vi "ControlRead.vi"(0 "Data input":T1, 1 "Selected Item":string[](array[string]), 5 "error in":errorcluster) -> (14 "Data output":T1, 19 "error out":errorcluster)   [LabVIEW 2017]
doc: "<B>This VI is used for getting the selelcted property type, value and index, and setting the control value.</B>"
uses:
  <vilib>/Utility/miscctls.llb/LVStringsAndValuesArrayTypeDef_U16.ctl
  API/Tree/SLSC Tree Control.lvlib
  <vilib>/JDP Science/JSONtext/JSONtext.lvlib
  cd6786a6-1ea5-437c-bd7d-10aa4f833b89.vi
  1b247805-81af-4051-83cb-4bfd180f6ea7.vi
  Ctrl/Property.ctl
  Ctrl/PhysicalChannel.ctl
  Ctrl/Bitfield.ctl
  Ctrl/Register.ctl
  Ctrl/ScaleType.ctl
  Ctrl/Scale.ctl
  Ctrl/EnumValue.ctl
  Ctrl/Enum.ctl
  Ctrl/Caps.ctl
  Ctrl/Data.ctl
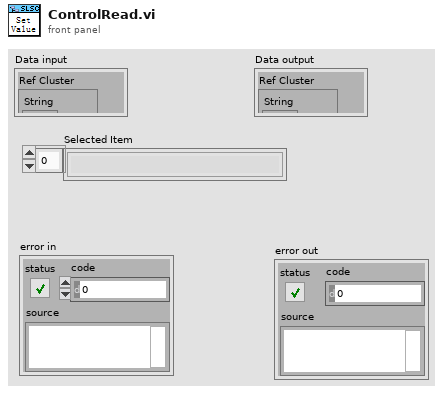
[diagram p1: front panel]
types:
  T1 = typedef "Data.ctl" = cluster{"Ref Cluster":cluster{"String":refnum<vi>, "U8":refnum<vi>, "I8":refnum<vi>, "U32":refnum<vi>, "I32":refnum<vi>, "U64":refnum<vi>, "I64":refnum<vi>, "Ring":refnum<vi>, "DBL":refnum<vi>, "Add":refnum<vi>, "Remove":refnum<vi>, "Property tree":refnum<vi>, "confirm":refnum<vi>}, "JSON Text":string, "Original JSON Text":string, "Caps":T2, "SLSC Output Tree":cluster{"Left Cell String":string, "Child Text":string[], "Child Tag":string, "Item Indent":i32, "Child Only?":bool, "Glyph Index":i32, "offline value":variant}[], "Ref Index and Control Type":cluster{"index":i32, "Datatype":string}, "Selected Type and name":cluster{"Selected Type":enum16{"Property", "Physical Channel", "Other"}, "Selected Property Name":string}, "Update whole Tree?":bool}
  T2 = typedef "Caps.ctl" = cluster{"properties":T3[], "physical channels":T4[], "registers":T5[], "scales":T7[], "enums":T9[], "productName":string}
  T3 = typedef "Property.ctl" = cluster{"name":string, "bitfield":string, "value":variant, "dataType":string, "min":variant, "max":variant, "scale":string, "access":string}
  T4 = typedef "PhysicalChannel.ctl" = cluster{"name":string, "properties":T3[]}
  T5 = typedef "Register.ctl" = cluster{"name":string, "address":i32, "size":i32, "bitfields":T6[], "initialValue":variant, "connectedProperties":string[]}
  T6 = typedef "Bitfield.ctl" = cluster{"name":string, "offset":i32, "size":i32, "signed":bool}
  T7 = typedef "Scale.ctl" = cluster{"name":string, "type":T8, "params":variant}
  T8 = typedef "ScaleType.ctl" = enum16{"NoScale", "Table", "Polynomial", "Linear"}
  T9 = typedef "Enum.ctl" = cluster{"name":string, "values":T10[]}
  T10 = typedef "EnumValue.ctl" = cluster{"name":string, "value":i32}
  T11 = enum16{"Show Selected Control", "All Visiable", "All Invisible"}
  T12 = cluster{"String":refnum<vi>, "U8":refnum<vi>, "I8":refnum<vi>, "U32":refnum<vi>, "I32":refnum<vi>, "U64":refnum<vi>, "I64":refnum<vi>, "Ring":refnum<vi>, "DBL":refnum<vi>, "Add":refnum<vi>, "Remove":refnum<vi>, "Property tree":refnum<vi>, "confirm":refnum<vi>}
  T13 = typedef "LVStringsAndValuesArrayTypeDef_U16.ctl" = cluster{"String":string, "Value":u16}[]
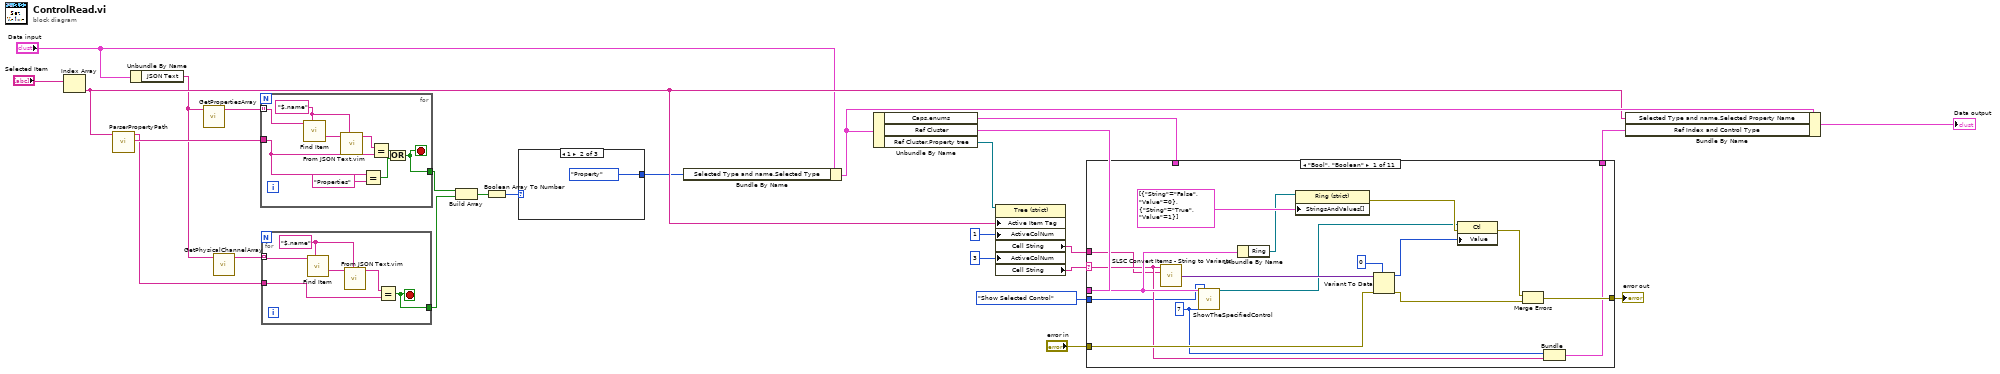
[diagram p0: block diagram]
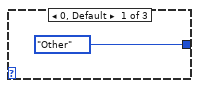
[diagram p2: hidden frame]
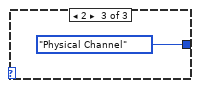
[diagram p3: hidden frame]
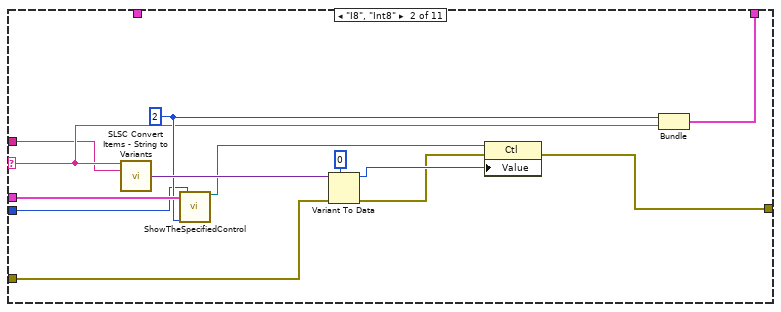
[diagram p4: hidden frame]
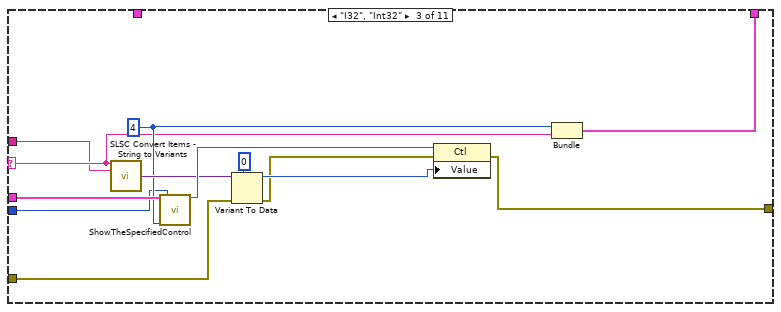
[diagram p5: hidden frame]
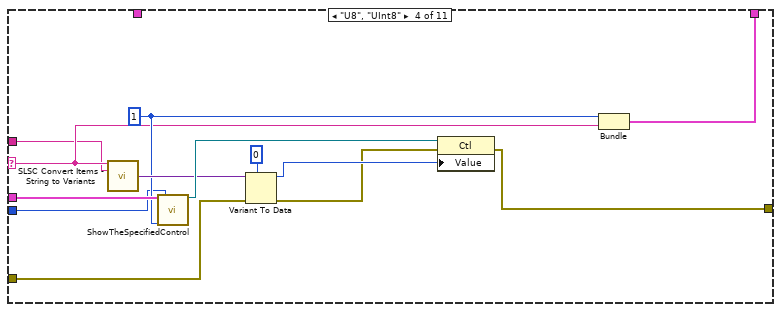
[diagram p6: hidden frame]
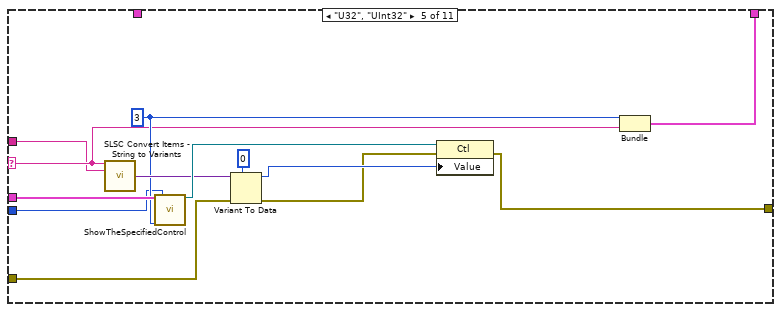
[diagram p7: hidden frame]
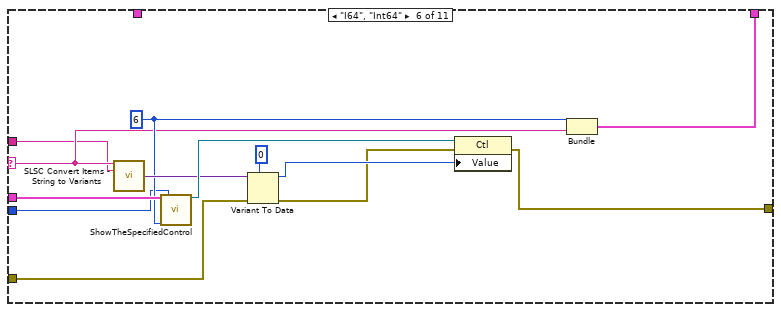
[diagram p8: hidden frame]
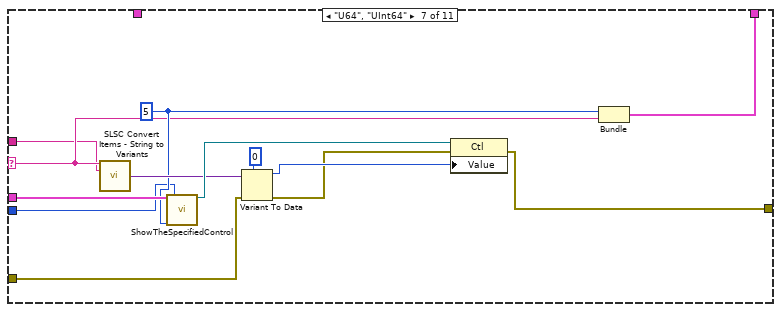
[diagram p9: hidden frame]
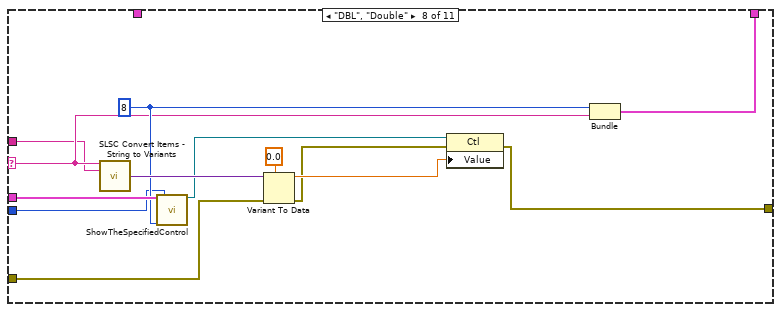
[diagram p10: hidden frame]
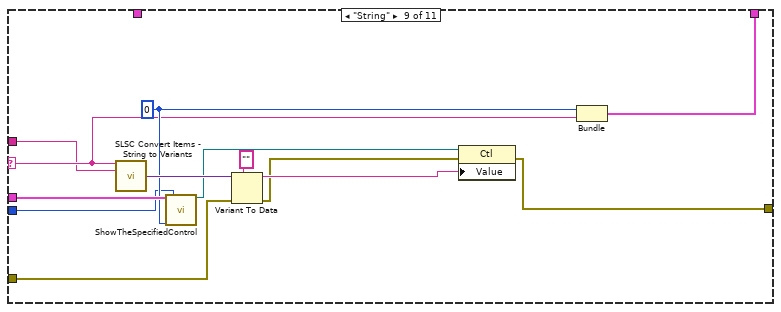
[diagram p11: hidden frame]
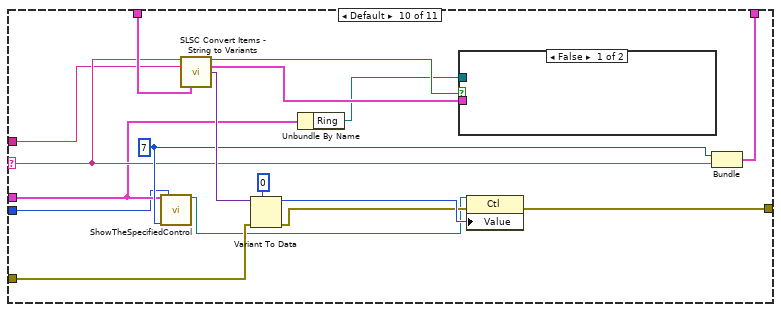
[diagram p12: hidden frame]
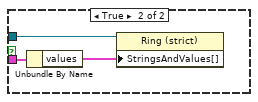
[diagram p13: hidden frame]
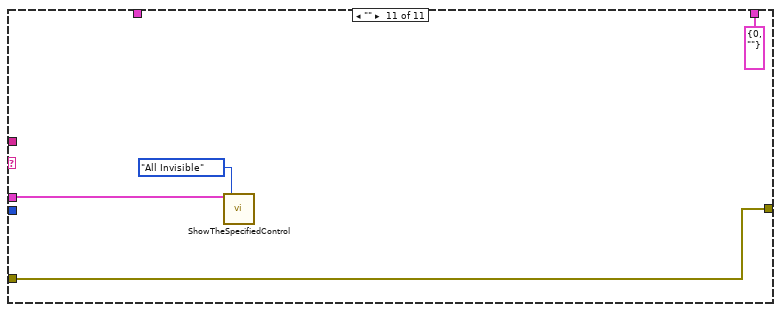
[diagram p14: hidden frame]
diagram:
  n1 = Index Array(array="Selected Item") -> (element=w13:string)  [unwired: 1 in]
  n2 = call "ParserPropertyPath.vi"("property"=w13) -> ("name"=w11:string, "pyhsical channel"=w8:string)  [unwired: 7 in]
  n3 = Unbundle By Name("Data input") -> ("JSON Text"=w10:string)
  n4 = call "GetPropertiesArray.vi"("JSON Text"=w10) -> ("Properties Array"=w12:string[])  [unwired: 9 in, 1 out]
  n5 = call "GetPhysicalChannelArray.vi"("JSON Text"=w10) -> ("PhysicalChannels Array"=w9:string[])  [unwired: 9 in, 1 out]
  n6 = for {
    tunnel: w12 -> [w35] mode=indexing
    tunnel: w11 -> [w28]
    tunnel: [w30] -> w7
    stop <- w30 stop-if-true
    w33 = "$.name" ("$Path or Item Name")
    n7 = call <vilib>:"Find Item.vi"("$Path or Item Name"=w33, "JSON"=w35) -> ("<JSON>"=w34:string)  [unwired: 6 in, 3 out]
    n8 = call "From JSON Text.vim"("Data Type and Default Value"=w33, "JSON"=w34) -> ("Data out"=w32:string)  [unwired: 8 in, 1 out]
    n9 = Equal?(x=w28, y="Properties") -> (x = y?=w29:bool)
    n10 = Equal?(x=w32, y=w28) -> (x = y?=w31:bool)
    n11 = Or(x=w31, y=w29) -> (x .or. y?=w30:bool)
  }
  n12 = for {
    tunnel: w9 -> [w41] mode=indexing
    tunnel: w8 -> [w37]
    tunnel: [w36] -> w6
    stop <- w36 stop-if-true
    w39 = "$.name" ("$Path or Item Name")
    n13 = call <vilib>:"Find Item.vi"("$Path or Item Name"=w39, "JSON"=w41) -> ("<JSON>"=w40:string)  [unwired: 6 in, 3 out]
    n14 = call "From JSON Text.vim"("Data Type and Default Value"=w39, "JSON"=w40) -> ("Data out"=w38:string)  [unwired: 8 in, 1 out]
    n15 = Equal?(x=w38, y=w37) -> (x = y?=w36:bool)
  }
  n16 = Build Array(w7, w6) -> (w5:bool[])
  n17 = Boolean Array To Number(Boolean array=w5) -> (number=w4:u32)
  n18 = case shown="1" w4 {
    tunnel: [enum16{"Property", "Physical Channel", "Other"}."Other" ("Selected Type and name.Selected Type") enum16{"Property", "Physical Channel", "Other"}."Property" ("Selected Type and name.Selected Type") enum16{"Property", "Physical Channel", "Other"}."Physical Channel" ("Selected Type and name.Selected Type")] -> w3
    frame 0, Default {
    }
    frame 1 {
    }
    frame 2 {
    }
  }
  n19 = Bundle By Name(cluster="Data input", "Selected Type and name.Selected Type"=w3) -> (w21:T1)
  n20 = Unbundle By Name(w21) -> ("Caps.enums"=w26:T9[], "Ref Cluster"=w25:T12, "Ref Cluster.Property tree"=w18:refnum<vi>)
  n21 = property class="Tree (strict)"(reference=w18, "Active Item Tag"=w13, "ActiveColNum"=1 ("Active Cell:Active Column Number"), "ActiveColNum"=3 ("Active Cell:Active Column Number")) -> ("Cell String"=w15:string, "Cell String"=w14:string)  [unwired: 1 in, 2 out]
  n22 = case shown="\"Bool\", \"Boolean\"" w14 {
    selector: w14 -> [w48 w65 w78 w91 w104 w117 w130 w143 w156 w171 _]
    tunnel: [w54 w69 w80 w93 w106 w119 w132 w145 w158 w174 w187] -> w22
    tunnel: "error in" -> [w55 w67 w82 w95 w108 w121 w134 w147 w160 w176 w187]
    tunnel: w26 -> [_ _ _ _ _ _ _ _ _ w177 _]
    tunnel: w25 -> [w51 w70 w83 w96 w109 w122 w135 w148 w161 w169 w186]
    tunnel: [w47 w64 w77 w90 w103 w116 w129 w142 w155 w170 cluster{"index":i32, string} {"index"=0, ""}] -> w23
    tunnel: w15 -> [w46 w63 w76 w89 w102 w115 w128 w141 w154 w167 _]
    tunnel: T11."Show Selected Control" ("Command") -> [w45 w62 w75 w88 w101 w114 w127 w140 w153 w166 _]
    frame "Bool", "Boolean" {
      w49 = 7 ("index")
      n23 = call "SLSC Convert Items - String to Variants.vi"("Datatype"=w48, "Value"=w46) -> ("Value"=w60:variant)  [unwired: 11 in, 2 out]
      n24 = call "ShowTheSpecifiedControl.vi"("Ref Cluster"=w51, "index"=w49, "Command"=w45) -> ("element"=w56:refnum<vi>)  [unwired: 16 in]
      n25 = Unbundle By Name(w51) -> ("Ring"=w50:refnum<vi>)
      n26 = property on="Property Node" class="Ring (strict)"(reference=w50, "StringsAndValues[]"=T13 [{"String"="False", "Value"=0}, {"String"="True", "Value"=1}] ("Strings And Values []")) -> (error out=w57:errorcluster)  [unwired: 1 in, 1 out]
      n27 = Variant To Data(error in=w55, type=u16 0 ("Value"), Variant=w60) -> (data=w59:u16, error out=w52:errorcluster)
      n28 = property class="Ctl"(reference=w56, error in=w57, "Value"=w59) -> (error out=w53:errorcluster)  [unwired: 1 out]
      n29 = Merge Errors(w53, w52) -> (w54:errorcluster)
      n30 = Bundle("index"=w49, w48) -> (w47:cluster{"index":i32, string})  [unwired: 1 in]
    }
    frame "I8", "Int8" {
      w66 = 2 ("index")
      n31 = call "SLSC Convert Items - String to Variants.vi"("Datatype"=w65, "Value"=w63) -> ("Value"=w73:variant)  [unwired: 11 in, 2 out]
      n32 = call "ShowTheSpecifiedControl.vi"("Ref Cluster"=w70, "index"=w66, "Command"=w62) -> ("element"=w71:refnum<vi>)  [unwired: 16 in]
      n33 = Variant To Data(error in=w67, type=i8 0 ("Value"), Variant=w73) -> (data=w72:i8, error out=w68:errorcluster)
      n34 = property class="Ctl"(reference=w71, error in=w68, "Value"=w72) -> (error out=w69:errorcluster)  [unwired: 1 out]
      n35 = Bundle("index"=w66, w65) -> (w64:cluster{"index":i32, string})  [unwired: 1 in]
    }
    frame "I32", "Int32" {
      w79 = 4 ("index")
      n36 = call "SLSC Convert Items - String to Variants.vi"("Datatype"=w78, "Value"=w76) -> ("Value"=w84:variant)  [unwired: 11 in, 2 out]
      n37 = call "ShowTheSpecifiedControl.vi"("Ref Cluster"=w83, "index"=w79, "Command"=w75) -> ("element"=w86:refnum<vi>)  [unwired: 16 in]
      n38 = Variant To Data(error in=w82, type=0 ("Value"), Variant=w84) -> (data=w85:i32, error out=w81:errorcluster)
      n39 = property class="Ctl"(reference=w86, error in=w81, "Value"=w85) -> (error out=w80:errorcluster)  [unwired: 1 out]
      n40 = Bundle("index"=w79, w78) -> (w77:cluster{"index":i32, string})  [unwired: 1 in]
    }
    frame "U8", "UInt8" {
      w92 = 1 ("index")
      n41 = call "SLSC Convert Items - String to Variants.vi"("Datatype"=w91, "Value"=w89) -> ("Value"=w97:variant)  [unwired: 11 in, 2 out]
      n42 = call "ShowTheSpecifiedControl.vi"("Ref Cluster"=w96, "index"=w92, "Command"=w88) -> ("element"=w99:refnum<vi>)  [unwired: 16 in]
      n43 = Variant To Data(error in=w95, type=u8 0 ("Value"), Variant=w97) -> (data=w98:u8, error out=w94:errorcluster)
      n44 = property class="Ctl"(reference=w99, error in=w94, "Value"=w98) -> (error out=w93:errorcluster)  [unwired: 1 out]
      n45 = Bundle("index"=w92, w91) -> (w90:cluster{"index":i32, string})  [unwired: 1 in]
    }
    frame "U32", "UInt32" {
      w105 = 3 ("index")
      n46 = call "SLSC Convert Items - String to Variants.vi"("Datatype"=w104, "Value"=w102) -> ("Value"=w110:variant)  [unwired: 11 in, 2 out]
      n47 = call "ShowTheSpecifiedControl.vi"("Ref Cluster"=w109, "index"=w105, "Command"=w101) -> ("element"=w112:refnum<vi>)  [unwired: 16 in]
      n48 = Variant To Data(error in=w108, type=u32 0 ("Value"), Variant=w110) -> (data=w111:u32, error out=w107:errorcluster)
      n49 = property class="Ctl"(reference=w112, error in=w107, "Value"=w111) -> (error out=w106:errorcluster)  [unwired: 1 out]
      n50 = Bundle("index"=w105, w104) -> (w103:cluster{"index":i32, string})  [unwired: 1 in]
    }
    frame "I64", "Int64" {
      w118 = 6 ("index")
      n51 = call "SLSC Convert Items - String to Variants.vi"("Datatype"=w117, "Value"=w115) -> ("Value"=w123:variant)  [unwired: 11 in, 2 out]
      n52 = call "ShowTheSpecifiedControl.vi"("Ref Cluster"=w122, "index"=w118, "Command"=w114) -> ("element"=w125:refnum<vi>)  [unwired: 16 in]
      n53 = Variant To Data(error in=w121, type=i64 0 ("Value"), Variant=w123) -> (data=w124:i64, error out=w120:errorcluster)
      n54 = property class="Ctl"(reference=w125, error in=w120, "Value"=w124) -> (error out=w119:errorcluster)  [unwired: 1 out]
      n55 = Bundle("index"=w118, w117) -> (w116:cluster{"index":i32, string})  [unwired: 1 in]
    }
    frame "U64", "UInt64" {
      w131 = 5 ("index")
      n56 = call "SLSC Convert Items - String to Variants.vi"("Datatype"=w130, "Value"=w128) -> ("Value"=w136:variant)  [unwired: 11 in, 2 out]
      n57 = call "ShowTheSpecifiedControl.vi"("Ref Cluster"=w135, "index"=w131, "Command"=w127) -> ("element"=w138:refnum<vi>)  [unwired: 16 in]
      n58 = Variant To Data(error in=w134, type=u64 0, Variant=w136) -> (data=w137:u64, error out=w133:errorcluster)
      n59 = property class="Ctl"(reference=w138, error in=w133, "Value"=w137) -> (error out=w132:errorcluster)  [unwired: 1 out]
      n60 = Bundle("index"=w131, w130) -> (w129:cluster{"index":i32, string})  [unwired: 1 in]
    }
    frame "DBL", "Double" {
      w144 = 8 ("index")
      n61 = call "SLSC Convert Items - String to Variants.vi"("Datatype"=w143, "Value"=w141) -> ("Value"=w150:variant)  [unwired: 11 in, 2 out]
      n62 = call "ShowTheSpecifiedControl.vi"("Ref Cluster"=w148, "index"=w144, "Command"=w140) -> ("element"=w149:refnum<vi>)  [unwired: 16 in]
      n63 = Variant To Data(error in=w147, type=0.0 ("Value"), Variant=w150) -> (data=w151:dbl, error out=w146:errorcluster)
      n64 = property class="Ctl"(reference=w149, error in=w146, "Value"=w151) -> (error out=w145:errorcluster)  [unwired: 1 out]
      n65 = Bundle("index"=w144, w143) -> (w142:cluster{"index":i32, string})  [unwired: 1 in]
    }
    frame "String" {
      w157 = 0 ("index")
      n66 = call "SLSC Convert Items - String to Variants.vi"("Datatype"=w156, "Value"=w154) -> ("Value"=w163:variant)  [unwired: 11 in, 2 out]
      n67 = call "ShowTheSpecifiedControl.vi"("Ref Cluster"=w161, "index"=w157, "Command"=w153) -> ("element"=w162:refnum<vi>)  [unwired: 16 in]
      n68 = Variant To Data(error in=w160, type="" ("Value"), Variant=w163) -> (data=w164:string, error out=w159:errorcluster)
      n69 = property class="Ctl"(reference=w162, error in=w159, "Value"=w164) -> (error out=w158:errorcluster)  [unwired: 1 out]
      n70 = Bundle("index"=w157, w156) -> (w155:cluster{"index":i32, string})  [unwired: 1 in]
    }
    frame Default {
      w172 = 7 ("index")
      n71 = call "ShowTheSpecifiedControl.vi"("Ref Cluster"=w169, "index"=w172, "Command"=w166) -> ("element"=w173:refnum<vi>)  [unwired: 16 in]
      n72 = call "SLSC Convert Items - String to Variants.vi"("Datatype"=w171, "Value"=w167, "enums"=w177) -> ("Datatype found?"=w178:bool, "enum"=w179:T9, "Value"=w181:variant)  [unwired: 10 in]
      n73 = Variant To Data(error in=w176, type=0 ("Value"), Variant=w181) -> (data=w180:i32, error out=w175:errorcluster)
      n74 = Unbundle By Name(w169) -> ("Ring"=w168:refnum<vi>)
      n75 = case shown="False" w178 {
        tunnel: w179 -> [_ w185]
        tunnel: w168 -> [_ w183]
        frame False {
        }
        frame True {
          n76 = Unbundle By Name(w185) -> ("values"=w184:T10[])
          n77 = property on="Property Node" class="Ring (strict)"(reference=w183, "StringsAndValues[]"=w184) -> ()  [unwired: 1 in, 2 out]
        }
      }
      n78 = property class="Ctl"(reference=w173, error in=w175, "Value"=w180) -> (error out=w174:errorcluster)  [unwired: 1 out]
      n79 = Bundle("index"=w172, w171) -> (w170:cluster{"index":i32, string})  [unwired: 1 in]
    }
    frame "" {
      n80 = call "ShowTheSpecifiedControl.vi"("Ref Cluster"=w186, "Command"=T11."All Invisible") -> ()  [unwired: 17 in, 1 out]
    }
  }
  "error out" <- w22
  n81 = Bundle By Name(cluster=w21, "Selected Type and name.Selected Property Name"=w13, "Ref Index and Control Type"=w23) -> (→"Data output":T1)
